vi "TMC module control.vi"(2 "Nur Position auslesen":bool=TRUE, 3 "Winkel [°]":dbl min=-360.0 max=360.0 step=0.1, 4 "flow control":u16(ring) items=["None"=0, "XON/XOFF"=1, "RTS/CTS"=2, "DTR/DSR"=4], 5 "VISA resource name":refnum<visa-resource-name>="COM6", 6 "stop bits":u16(ring)=10 items=["1.0"=10, "1.5"=15, "2.0"=20], 7 "parity":u16(ring) items=["None", "Odd", "Even", "Mark", "Space"], 8 "data bits":u16=8 min=5 max=8 step=1, 9 "baud rate":u32=9600) -> (0 "Ausgelesener Winkel [°]":dbl format="%.1f", 1 "Fehler":bool)   [LabVIEW 2016]
doc: "Diese VI steuert einen Steppermotor mit TMCM-110 Modul.\nBei Start laufen folgende Schritte ab:\n1. Wenn \"nur Position auslesen\" deaktiviert ist\n- Überprüfe, ob neu gestartet wurde\n- falls ja: korregiere aktuelle Position auf letze Positionskoordinate vor Abschaltung\n- sende anzufahrende Position (Motor setzt sich in Bewegung)\n- Speichere neue Positions-Koordinate\n- lese aktuelle Position\n2. Wenn \"nur Position auslesen\" aktiviert\n- lese aktuelle Position\n\nDiese VI sollte nur ausgeführt werden, wenn vorher die VI \"Modul Reset\" auf den Motor\nausgeführt wurde"
uses:
  <vilib>/Instr/_visa.llb/VISA Configure Serial Port (Serial Instr).vi
panel:
  out "Schritte je Winkelgrad":dbl
  out "Auslgelesenes Array":u8[](array[numeric])
  out "Ausgegebener Wert\ndezimal":i32
  out "Type":string
  out "Data to write":string
  out "Instruction":string
  out "Motor":string
  out "Value":string
  # "Diese VI steuert einen Steppermotor mit TMCM-110 Modul.\nBei Start laufen folgende Schritte ab:\n1. Wenn \"nur Position auslesen\" deaktiviert ist\n- Überprüfe, ob neu gestartet wurde\n- falls ja: korregiere aktuelle Position auf letze Positionskoordinate vor Abschaltung\n- sende anzufahrende Position (Motor setzt sich in Bewegung)\n- Speichere neue Positions-Koordinate\n- lese aktuelle Position\n2. Wenn \"nur Position auslesen\" aktiviert\n- lese aktuelle Position\n\nDiese VI sollte nur ausgeführt werden, wenn vorher ein mal die VI \"Modul Reset\" auf den Motor\nausgeführt wurde"
  # "RS232 configuration"
  # "Winkel Eingabe und Auslese"
  # "Kontrolldaten"
  # "Leuchtet diese Lampe auf kann der Motor nicht ausgelesen werden!\nFolgende Ursachen sind möglich:\n-Motor hat keinen Strom\n-Motor ist nicht angeschlossen\n-RS232 Konfigurationen sind falsch"
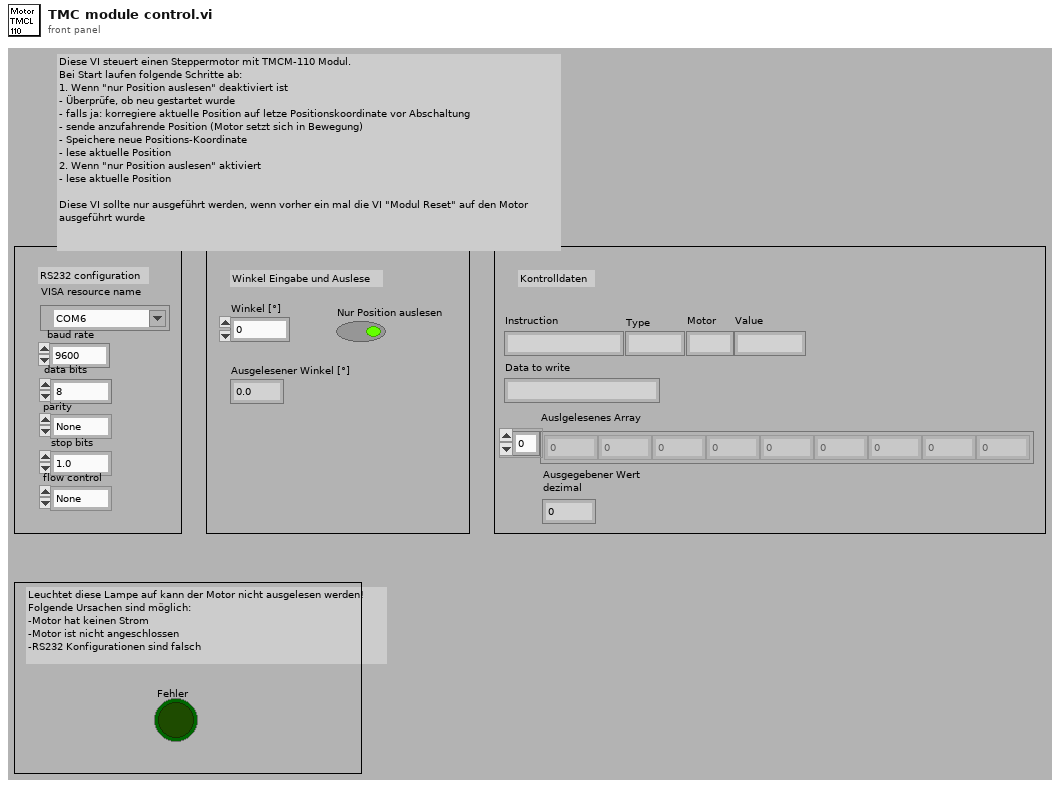
[diagram p1: front panel]
types:
  T1 = cluster{"Laufnummer":i32, "Aktuelle Position":i32, "Zielposition":i32, "gespeicherte Kooridnate":i32, "Case \"Neustart\"":bool}
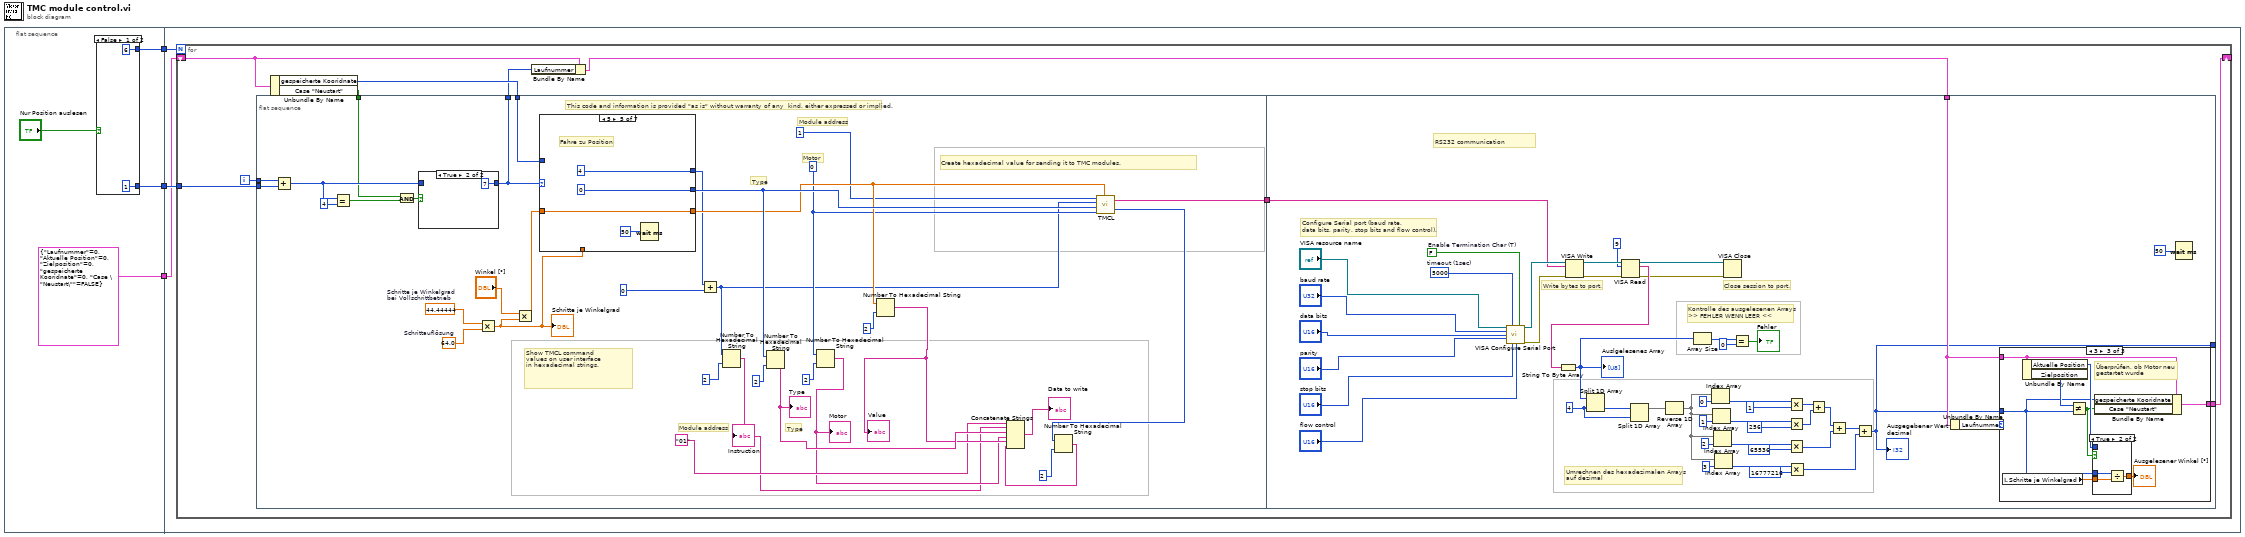
[diagram p0: block diagram]
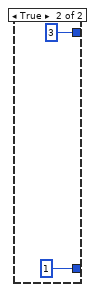
[diagram p2: hidden frame]
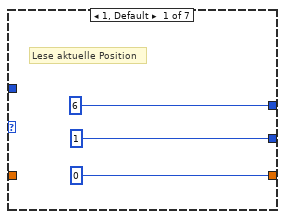
[diagram p4: hidden frame]
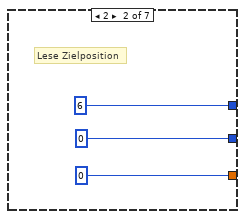
[diagram p5: hidden frame]
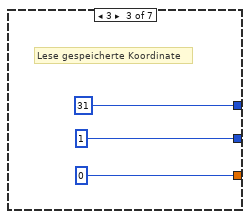
[diagram p6: hidden frame]
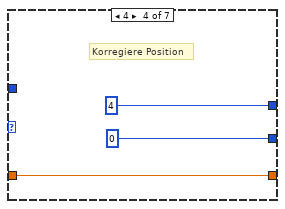
[diagram p7: hidden frame]
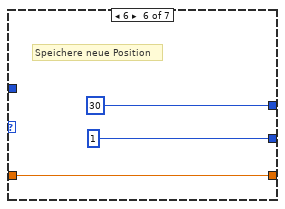
[diagram p8: hidden frame]
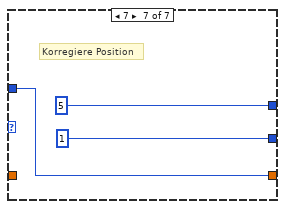
[diagram p9: hidden frame]
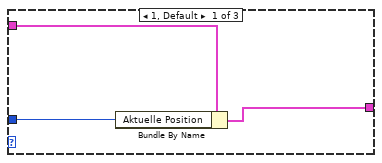
[diagram p10: hidden frame]
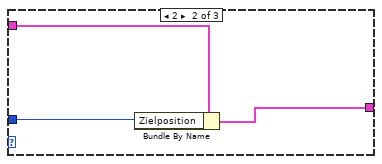
[diagram p11: hidden frame]
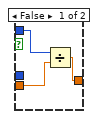
[diagram p12: hidden frame]
diagram:
  n1 = flat-sequence {
    tunnel: [w7] -> w3
    tunnel: [w5] -> w2
    tunnel: [T1 {"Laufnummer"=0, "Aktuelle Position"=0, "Zielposition"=0, "gespeicherte Kooridnate"=0, "Case \"Neustart\""=FALSE}] -> w1
    tunnel: w3 -> [w14]
    tunnel: w2 -> [w13]
    tunnel: w1 -> [w12]
    frame #0 {
      n2 = case shown="False" "Nur Position auslesen" {
        tunnel: [1 ("y") 1 ("y")] -> w7
        tunnel: [6 3] -> w5
        frame False {
        }
        frame True {
        }
      }
    }
    frame #1 {
      n3 = for {
        N: w13 -> [_]
        tunnel: w14 -> [w22]
        shift-right: [w20] -> _
        shift-left: w12 -> [w18]
        i -> [w23]
        n4 = flat-sequence {
          tunnel: w23 -> [w30]
          tunnel: [w38] -> w21
          tunnel: w22 -> [w36]
          tunnel: w19 -> [w32]
          tunnel: [w27] -> w16
          tunnel: w15 -> [w25]
          tunnel: [w88] -> _
          tunnel: w21 -> [w120]
          tunnel: w17 -> [w89]
          tunnel: [w87] -> w20
          frame #0 {
            w33 = 64.0  # Schrittauflösung
            w34 = 44.44444  # Schritte je Winkelgrad bei Vollschrittbetrieb
            w54 = 0 ("Motor")
            # "Motor"
            # "Type"
            # "This code and information is provided \"as is\" without warranty of any  kind, either expressed or implied."
            # "Create hexadecimal value for sending it to TMC modules."
            # "Show TMCL command\nvalues on user interface\nin hexadecimal strings."
            # "Type"
            # "Module address"
            # "Module address"
            n5 = Add(x=w30, y=w36) -> (x+y=w28:i32)
            n6 = Equal?(x=w28, y=4) -> (x = y?=w24:bool)
            n7 = And(x=w25, y=w24) -> (x .and. y?=w26:bool)
            n8 = case shown="True" w26 {
              tunnel: w28 -> [w59 _]
              tunnel: [w59 7] -> w27
              frame False {
              }
              frame True {
              }
            }
            n9 = Multiply(x=w34, y=w33) -> (x*y=w31:dbl)
            "Schritte je Winkelgrad" <- w31
            n10 = Multiply(x="Winkel [°]", y=w31) -> (x*y=w37:dbl)
            n11 = case shown="5" w27 {
              tunnel: [6 6 31 4 4 30 5] -> w53
              tunnel: [1 0 1 0 0 1 1] -> w57
              tunnel: [0 0 0 w70 w74 w77 w80] -> w55
              tunnel: w37 -> [_ _ _ w70 w74 w77 _]
              tunnel: w32 -> [_ _ _ _ _ _ w80]
              tunnel: w31 -> [_ _ _ _ _ _ _]
              frame 1, Default {
                # "Lese aktuelle Position"
              }
              frame 2 {
                # "Lese Zielposition"
              }
              frame 3 {
                # "Lese gespeicherte Koordinate"
              }
              frame 4 {
                # "Korregiere Position"
              }
              frame 5 {
                # "Fahre zu Position"
                n12 = Wait (ms)(milliseconds to wait=u32 50 ("Zu wartende ms")) -> ()  [unwired: 1 out]
              }
              frame 6 {
                # "Speichere neue Position"
              }
              frame 7 {
                # "Korregiere Position"
              }
            }
            n13 = Add(x=w53, y=0) -> (x+y=w48:i32)
            n14 = Number To Hexadecimal String(1:2, 2:w48) -> (0:w41:string)
            "Instruction" <- w41
            n15 = Number To Hexadecimal String(1:2, 2:w57) -> (0:w58:string)
            "Type" <- w58
            n16 = Number To Hexadecimal String(1:2, 2:w54) -> (0:w44:string)
            "Motor" <- w44
            n17 = Number To Hexadecimal String(1:2, 2:w55) -> (0:w51:string)
            "Value" <- w51
            n18 = call "TMCL.vi"("Address"=1, "Instruction"=w48, "Type"=w57, "Motor"=w54, "Value"=w55) -> ("Hexadecimal value"=w38:string, "CRC (Optional)"=w52:i32)
            n19 = Number To Hexadecimal String(1:2, 2:w52) -> (0:w47:string)
            n20 = Concatenate Strings("01", w41, w58, w44, w51, w47) -> (→"Data to write":string)
          }
          frame #1 {
            w111 = 4 ("Index")
            w122 = FALSE  # Enable Termination Char (T)
            w121 = u32 5000  # timeout (1sec)
            # "Umrechnen des hexadezimalen Arrays\nauf dezimal"
            # "Kontrolle des ausgelesenen Arrays\n>> FEHLER WENN LEER <<"
            # "RS232 communication"
            # "Write bytes to port."
            # "Configure Serial port (baud rate,\ndata bits, parity, stop bits and flow control)."
            # "Close session to port."
            n21 = call-poly "VISA Configure Serial Port"("VISA resource name"="VISA resource name", "timeout (10sec)"=w121, "Enable Termination\nChar (T)"=w122, "baud rate (9600)"="baud rate", "data bits (8)"="data bits", "parity (0:none)"="parity", "stop bits (10: 1 bit)"="stop bits", "flow control (0:none)"="flow control") -> ("VISA resource name out"=w129:refnum<visa-resource-name>, "error out"=w130:errorcluster)  [unwired: 6 in]
            n22 = VISA Write(VISA resource name=w129, write buffer=w120, error in (no error)=w130) -> (VISA resource name out=w115:refnum<visa-resource-name>, error out=w114:errorcluster)  [unwired: 1 out]
            n23 = VISA Read(VISA resource name=w115, byte count=u32 9 ("General Settings:Timeout Value"), error in (no error)=w114) -> (VISA resource name out=w118:refnum<visa-resource-name>, read buffer=w119:string, error out=w117:errorcluster)  [unwired: 1 out]
            n24 = String To Byte Array(string=w119) -> (unsigned byte array=w86:u8[])
            "Auslgelesenes Array" <- w86
            n25 = Split 1D Array(array=w86, index=w111) -> (second subarray=w112:u8[])  [unwired: 1 out]
            n26 = Split 1D Array(array=w112, index=w111) -> (first subarray=w91:u8[])  [unwired: 1 out]
            n27 = Reverse 1D Array(array=w91) -> (reversed array=w105:u8[])
            n28 = Array Size(array=w86) -> (size(s)=w85:i32)
            n29 = Index Array(array=w105, index=0 ("Index")) -> (element=w101:u8)
            n30 = Index Array(array=w105, index=1 ("Index")) -> (element=w100:u8)
            n31 = Index Array(array=w105, index=2 ("Index")) -> (element=w99:u8)
            n32 = Index Array(array=w105, index=3 ("Index")) -> (element=w98:u8)
            n33 = VISA Close(VISA resource name=w118, error in (no error)=w117) -> ()  [unwired: 1 out]
            n34 = Equal?(x=w85, y=0) -> (x = y?=→"Fehler":bool)
            n35 = Multiply(x=w101, y=1) -> (x*y=w97:i32)
            n36 = Multiply(x=w100, y=256) -> (x*y=w96:i32)
            n37 = Multiply(x=w99, y=65536) -> (x*y=w94:i32)
            n38 = Multiply(x=w98, y=16777216) -> (x*y=w93:i32)
            n39 = Add(x=w97, y=w96) -> (x+y=w95:i32)
            n40 = Add(x=w95, y=w94) -> (x+y=w92:i32)
            n41 = Add(x=w92, y=w93) -> (x+y=w88:i32)
            "Ausgegebener Wert\ndezimal" <- w88
            n42 = Unbundle By Name(w89) -> ("Laufnummer"=w90:i32)
            n43 = case shown="3" w90 {
              tunnel: w89 -> [w133 w136 w141]
              tunnel: [w132 w135 w140] -> w87
              tunnel: w88 -> [w131 w134 w138]
              frame 1, Default {
                n44 = Bundle By Name(cluster=w133, "Aktuelle Position"=w131) -> (w132:T1)
              }
              frame 2 {
                n45 = Bundle By Name(cluster=w136, "Zielposition"=w134) -> (w135:T1)
              }
              frame 3 {
                # "Überprüfen, ob Motor neu\ngestartet wurde"
                n46 = local read "Schritte je Winkelgrad"() -> (w144:dbl)
                n47 = Unbundle By Name(w141) -> ("Aktuelle Position"=w143:i32, "Zielposition"=w139:i32)
                n48 = Not Equal?(x=w139, y=w138) -> (x != y?=w137:bool)
                n49 = case shown="True" w137 {
                  tunnel: w143 -> [w147 _]
                  tunnel: w138 -> [_ w150]
                  tunnel: [w146 w149] -> w142
                  tunnel: w144 -> [w145 w148]
                  frame False {
                    n50 = Divide(x=w147, y=w145) -> (x/y=w146:dbl)
                  }
                  frame True {
                    n51 = Divide(x=w150, y=w148) -> (x/y=w149:dbl)
                  }
                }
                "Ausgelesener Winkel [°]" <- w142
                n52 = Bundle By Name(cluster=w141, "gespeicherte Kooridnate"=w138, "Case \"Neustart\""=w137) -> (w140:T1)
              }
            }
            n53 = Wait (ms)(milliseconds to wait=u32 50 ("Zu wartende ms")) -> ()  [unwired: 1 out]
          }
        }
        n54 = Unbundle By Name(w18) -> ("gespeicherte Kooridnate"=w19:i32, "Case \"Neustart\""=w15:bool)
        n55 = Bundle By Name(cluster=w18, "Laufnummer"=w16) -> (w17:T1)
      }
    }
  }
